vi "Connect_Open.vi"(8 "error in (no error)":errorcluster, 11 "VISA Refnum in":refnum<visa-resource-name>) -> (0 "error out":errorcluster, 3 "VISA Refnum out":refnum<visa-resource-name>)   [LabVIEW 2019]
uses:
  ef00ffa6-4583-4add-bc54-34e85376bb40.vi
  13994e47-8e2a-4767-a9f4-097228dc03a3.vi
  <vilib>/Instr/_visa.llb/VISA Configure Serial Port (Instr).vi
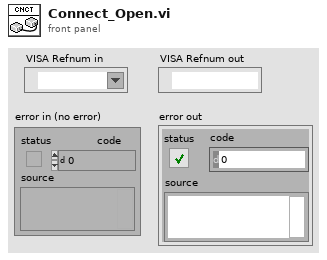
[diagram p1: front panel]
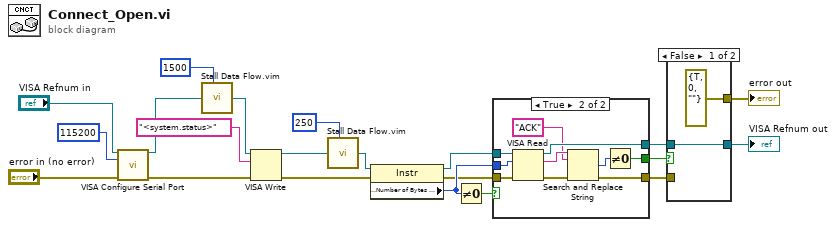
[diagram p0: block diagram]
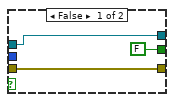
[diagram p2: hidden frame]
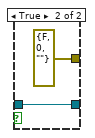
[diagram p3: hidden frame]
diagram:
  n1 = call-poly "VISA Configure Serial Port"("VISA resource name"="VISA Refnum in", "baud rate (9600)"=u32 115200, "error in (no error)"="error in (no error)") -> ("VISA resource name out"=w18:refnum<visa-resource-name>, "error out"=w19:errorcluster)  [unwired: 11 in]
  n2 = call "Stall Data Flow.vim"("value in"=w18, "milliseconds to wait"=u32 1500) -> ("value out"=w16:refnum<visa-resource-name>)  [unwired: 1 out]
  n3 = VISA Write(VISA resource name=w16, write buffer="<system.status>", error in (no error)=w19) -> (VISA resource name out=w4:refnum<visa-resource-name>, error out=w5:errorcluster)  [unwired: 1 out]
  n4 = call "Stall Data Flow.vim"("value in"=w4, "milliseconds to wait"=u32 250) -> ("value out"=w13:refnum<visa-resource-name>)  [unwired: 1 out]
  n5 = property class="Instr"(reference=w13, error in=w5) -> (reference out=w7:refnum<visa-resource-name>, error out=w8:errorcluster, "Serial Settings:Number of Bytes at Serial Port"=w12:u32)
  n6 = Not Equal To 0?(x=w12) -> (x != 0?=w6:bool)
  n7 = case shown="True" w6 {
    tunnel: [w24 w34] -> w10
    tunnel: w7 -> [w24 w33]
    tunnel: w12 -> [_ w32]
    tunnel: [FALSE w28] -> w9
    tunnel: w8 -> [w22 w27]
    tunnel: [w22 w25] -> w11
    frame False {
    }
    frame True {
      n8 = VISA Read(VISA resource name=w33, byte count=w32, error in (no error)=w27) -> (VISA resource name out=w34:refnum<visa-resource-name>, read buffer=w30:string, error out=w26:errorcluster)  [unwired: 1 out]
      n9 = Search and Replace String(input string=w30, search string="ACK", error in=w26) -> (number of replacements=w31:i32, error out=w25:errorcluster)  [unwired: 5 in, 2 out]
      n10 = Not Equal To 0?(x=w31) -> (x != 0?=w28:bool)
    }
  }
  n11 = case shown="False" w9 {
    tunnel: w10 -> [w35 w37]
    tunnel: w11 -> [_ _]
    tunnel: [errorcluster {"status"=TRUE, "code"=0, "source"=""} ("error out") errorcluster {"status"=FALSE, "code"=0, "source"=""} ("error out")] -> w21
    tunnel: [w35 w37] -> w20
    frame False {
    }
    frame True {
    }
  }
  "error out" <- w21
  "VISA Refnum out" <- w20
